vi "Remote Calibration FPGA Loop.vi"   [LabVIEW 2014]
uses:
  Global Data.vi
  <vilib>/rvi/interface/nirviOpenFPGA/nirviOpenFPGA.xnode
  FPGA Bitfiles/FormulaElectric2_FPGATarget_FPGA_8a5J0mMac2U.lvbitx
  <vilib>/rvi/interface/nirviReadWriteControl/nirviReadWriteControl.xnode
  <vilib>/rvi/interface/Simulation/niFpgaSimulationCallBeginRW.vi
  <vilib>/rvi/errors/niLvFpgaAdjustHostInterfaceError.vi
  <vilib>/rvi/interface/nirviCloseFPGA/nirviCloseFPGA.xnode
  MC State Machine.lvsc/State.ctl
  MC State Machine.lvsc
  Remote Calibration Variable.vi
  Remote Calibration Typedef.ctl
  <vilib>/FPGAPlugInAG/sbRIO-9626/niLvFpga_Open_sbRIO-9626.vi
  <vilib>/rvi/interface/common/dynamic/niFpgaDynamicAddResources.vi
  <vilib>/FPGAPlugInAG/Dynamic/niLvFpga_Close_Dynamic.vi
types:
  T1 = typedef "Remote Calibration Typedef.ctl" = cluster{"Rear BP Scaling Factor":fxp<+,11,11>, "Front BP Scaling Factor":fxp<+,11,11>, "Rear BP Offset (V)":fxp<+/-,26,5>, "Front BP Offset":fxp<+/-,26,5>, "Throttle 2 Max":fxp<+,16,4>, "Throttle 2 Min":fxp<+,16,4>, "Throttle 1 Max":fxp<+,16,4>, "Throttle 1 Min":fxp<+,16,4>, "MC Update Period (ms)":u32, "Regen Mult.":dbl, "Zero Torque %":dbl, "Torque Mult.":dbl, "Activation Brake Pressure":dbl}
  T2 = typedef "MC State Machine.lvsc/State.ctl" = enum16{"NI.SC.Initial", "NI.SC.History", "NI.SC.ShallowHistory", "NI.SC.Terminal", "Let Current Drop then Disable AIR's", "Enabled", "Disabled"}
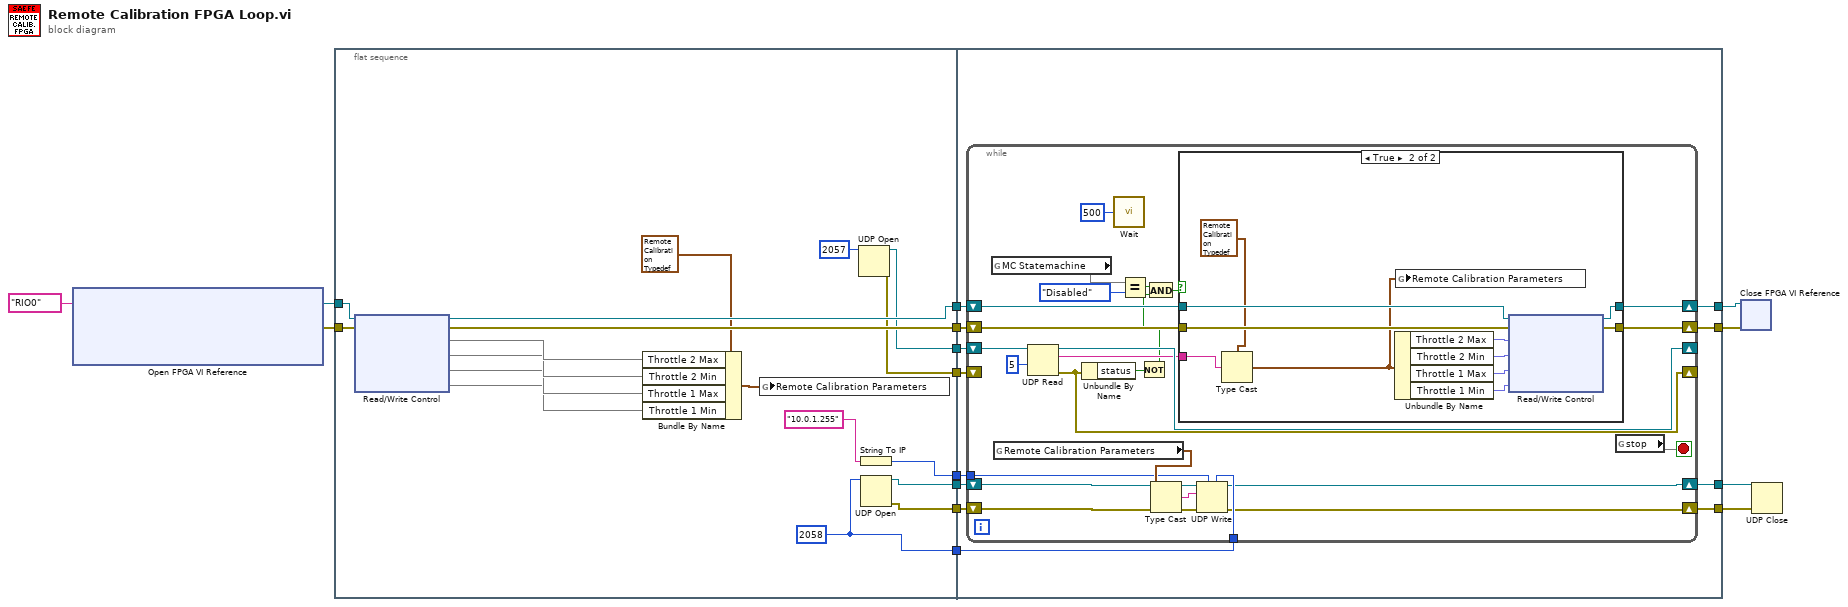
[diagram p0: block diagram]
diagram:
  n1 = xnode "Open FPGA VI Reference"("resource name"=tag "RIO0") -> ("FPGA VI Reference Out"=w15:refnum<k20>, "error out"=w14:errorcluster)  [unwired: 1 in]
  n2 = flat-sequence {
    tunnel: w15 -> [w33]
    tunnel: w14 -> [w32]
    tunnel: [w27] -> w13
    tunnel: [w26] -> w12
    tunnel: [w22] -> w8
    tunnel: [w21] -> w7
    tunnel: [w20] -> w6
    tunnel: [w19] -> w5
    tunnel: [w17] -> w2
    tunnel: [w16] -> w1
    tunnel: w13 -> [w45]
    tunnel: w12 -> [w44]
    tunnel: [w43] -> w11
    tunnel: [w42] -> w10
    tunnel: w8 -> [w41]
    tunnel: w7 -> [w40]
    tunnel: w6 -> [w39]
    tunnel: w5 -> [w38]
    tunnel: [w37] -> w4
    tunnel: [w36] -> w3
    tunnel: w2 -> [w35]
    tunnel: w1 -> [w34]
    frame #0 {
      w20 = u16 2058 ("port")
      n3 = xnode "Read/Write Control"("FPGA VI Reference In"=w33, "error in"=w32) -> ("FPGA VI Reference Out"=w27:refnum<k20>, "error out"=w26:errorcluster, "Throttle 2 Max"=w31, "Throttle 2 Min"=w30, "Throttle 1 Max"=w29, "Throttle 1 Min"=w28)
      n4 = Bundle By Name(cluster=T1 {"Rear BP Scaling Factor"=1250.0, "Front BP Scaling Factor"=1250.0, "Rear BP Offset (V)"=0.4820899963378906, "Front BP Offset"=0.4808177947998047, "Throttle 2 Max"=3.89990234375, "Throttle 2 Min"=2.090087890625, "Throttle 1 Max"=0.6298828125, "Throttle 1 Min"=2.4599609375, "MC Update Period (ms)"=20, "Regen Mult."=0.0, "Zero Torque %"=0.0, "Torque Mult."=160.0, "Activation Brake Pressure"=50.0} ("Remote Calibration Parameters"), "Throttle 2 Max"=w31, "Throttle 2 Min"=w30, "Throttle 1 Max"=w29, "Throttle 1 Min"=w28) -> (w25:T1)
      n5 = global write "Remote Calibration Variable.vi" "Remote Calibration Parameters"(w25) -> ()
      n6 = UDP Open(11:u16 2057 ("port")) -> (port=w17:refnum<k16>, 0:w16:errorcluster)  [unwired: 4 in, 1 out]
      n7 = String To IP(1:"10.0.1.255" ("name")) -> (0:w19:u32)
      n8 = UDP Open(11:w20) -> (port=w22:refnum<k16>, 0:w21:errorcluster)  [unwired: 4 in, 1 out]
    }
    frame #1 {
      n9 = while {
        shift-right: [w67] -> w43
        shift-left: w45 -> [w69]
        shift-right: [w66] -> w42
        shift-left: w44 -> [w68]
        tunnel: w39 -> [w59]
        tunnel: w38 -> [w58]
        shift-right: [w57] -> w37
        shift-left: w41 -> [w63]
        shift-right: [w56] -> w36
        shift-left: w40 -> [w62]
        shift-right: [w51] -> _
        shift-left: w35 -> [w53]
        shift-right: [w52] -> _
        shift-left: w34 -> [_]
        stop <- w70 stop-if-true
        n10 = global read "Global Data.vi" "MC Statemachine"() -> (w65)
        n11 = global read "Remote Calibration Variable.vi" "Remote Calibration Parameters"() -> (w60:T1)
        n12 = UDP Read(connection ID=w53, timeout ms (25000)=5) -> (data out=w50:string, error out=w52:errorcluster, 3:w51:refnum<k16>)  [unwired: 2 in, 2 out]
        n13 = Unbundle By Name(w52) -> ("status"=w48:bool)
        n14 = call "Wait"("Count(mSec)"=u32 500) -> ()  [unwired: 1 out]
        n15 = Equal?(x=w65, y=State."Disabled") -> (x = y?=w54:bool)
        n16 = Not(x=w48) -> (.not. x?=w47:bool)
        n17 = And(x=w54, y=w47) -> (x .and. y?=w55:bool)
        n18 = Type Cast(x=w60) -> (*(type *) &x=w61:string)  [unwired: 1 in]
        n19 = case shown="True" w55 {
          tunnel: w69 -> [w72 w83]
          tunnel: w68 -> [w71 w82]
          tunnel: [w72 w81] -> w67
          tunnel: [w71 w80] -> w66
          tunnel: w50 -> [_ w75]
          frame False {
          }
          frame True {
            n20 = Type Cast(type=T1 {"Rear BP Scaling Factor"=1250.0, "Front BP Scaling Factor"=1250.0, "Rear BP Offset (V)"=0.4820899963378906, "Front BP Offset"=0.4808177947998047, "Throttle 2 Max"=3.89990234375, "Throttle 2 Min"=2.090087890625, "Throttle 1 Max"=0.6298828125, "Throttle 1 Min"=2.4599609375, "MC Update Period (ms)"=20, "Regen Mult."=0.0, "Zero Torque %"=0.0, "Torque Mult."=160.0, "Activation Brake Pressure"=50.0} ("Remote Calibration Parameters"), x=w75) -> (*(type *) &x=w73:T1)
            n21 = Unbundle By Name(w73) -> ("Throttle 2 Max"=w79:fxp<+,16,4>, "Throttle 2 Min"=w78:fxp<+,16,4>, "Throttle 1 Max"=w77:fxp<+,16,4>, "Throttle 1 Min"=w76:fxp<+,16,4>)
            n22 = global write "Remote Calibration Variable.vi" "Remote Calibration Parameters"(w73) -> ()
            n23 = xnode "Read/Write Control"("FPGA VI Reference In"=w83, "error in"=w82, "Throttle 2 Max"=w79, "Throttle 2 Min"=w78, "Throttle 1 Max"=w77, "Throttle 1 Min"=w76) -> ("FPGA VI Reference Out"=w81:refnum<k20>, "error out"=w80:errorcluster)
          }
        }
        n24 = UDP Write(address=w58, port or service name=w59, connection ID=w63, data in=w61, 8:w62) -> (error out=w56:errorcluster, 3:w57:refnum<k16>)  [unwired: 1 in]
        n25 = global read "Global Data.vi" "stop"() -> (w70)
      }
    }
  }
  n26 = xnode "Close FPGA VI Reference"("FPGA VI Reference In"=w11, "error in"=w10) -> ()  [unwired: 1 out]
  n27 = UDP Close(connection ID=w4, 8:w3) -> ()  [unwired: 2 out]
